vi "checkData_priority.vi"(8 "error in (no error)":errorcluster, 9 "function return":i32, 10 "valExpect":i32, 11 "variant":variant) -> (0 "error out":errorcluster, 3 "isExpected":bool)   [LabVIEW 2018]
doc: "Check the data (priority)."
uses:
  VariantTool/getValFromVariant_I32.vi
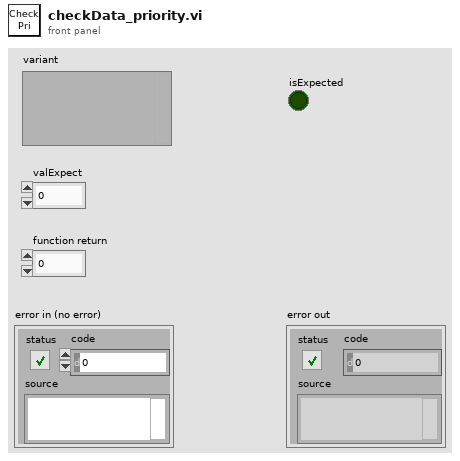
[diagram p1: front panel]
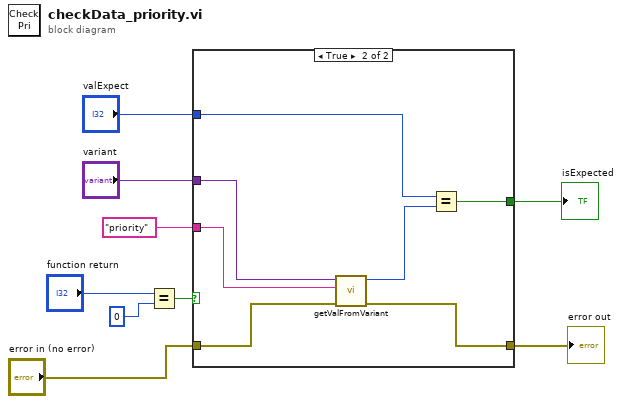
[diagram p0: block diagram]
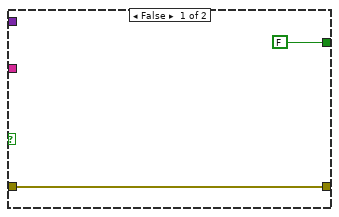
[diagram p2: hidden frame]
diagram:
  n1 = Equal?(x="function return", y=0 ("function return")) -> (x = y?=w8:bool)
  n2 = case shown="True" w8 {
    tunnel: "error in (no error)" -> [w11 w18]
    tunnel: [w11 w17] -> w5
    tunnel: "priority" ("name") -> [_ w16]
    tunnel: "variant" -> [_ w15]
    tunnel: "valExpect" -> [_ w14]
    tunnel: [FALSE w12] -> w1
    frame False {
    }
    frame True {
      n3 = call-poly "getValFromVariant.vi"("error in (no error)"=w18, "name"=w16, "variant"=w15) -> ("error out"=w17:errorcluster, "value"=w13:i32)  [unwired: 7 in]
      n4 = Equal?(x=w14, y=w13) -> (x = y?=w12:bool)
    }
  }
  "error out" <- w5
  "isExpected" <- w1
